vi "View Log Data.vi"() -> ()   [LabVIEW 2025]
uses:
  db86f9a9-b958-4c49-905b-a30c40e93e85.vi
  db86f9a9-b958-4c49-905b-a30c40e93e85.vi/4611cae3-c7be-41e2-9a5e-ea0ae78a7ced.vi
  db86f9a9-b958-4c49-905b-a30c40e93e85.vi/4611cae3-c7be-41e2-9a5e-ea0ae78a7ced.vi/19e2e4cb-e3bb-4239-bd5f-680916605f5d.vi
  db86f9a9-b958-4c49-905b-a30c40e93e85.vi/4611cae3-c7be-41e2-9a5e-ea0ae78a7ced.vi/f72612c1-738a-48a1-9fcf-3db66cb27fb3.vi
  db86f9a9-b958-4c49-905b-a30c40e93e85.vi/4611cae3-c7be-41e2-9a5e-ea0ae78a7ced.vi/45406051-8994-464b-8b47-ac12a8cbadfa.vi
  db86f9a9-b958-4c49-905b-a30c40e93e85.vi/4611cae3-c7be-41e2-9a5e-ea0ae78a7ced.vi/dd886480-778c-48b1-8e4a-d6890e1a60dd.vi
  db86f9a9-b958-4c49-905b-a30c40e93e85.vi/4611cae3-c7be-41e2-9a5e-ea0ae78a7ced.vi/2e6e140f-e361-4312-a09e-e37273ac7fd1.vi
  db86f9a9-b958-4c49-905b-a30c40e93e85.vi/4611cae3-c7be-41e2-9a5e-ea0ae78a7ced.vi/3589548e-4c68-4568-af05-72ab28470577.vi
  db86f9a9-b958-4c49-905b-a30c40e93e85.vi/4611cae3-c7be-41e2-9a5e-ea0ae78a7ced.vi/cf64d4f5-91bd-4749-9577-68c6ded0155b.vi
  db86f9a9-b958-4c49-905b-a30c40e93e85.vi/4611cae3-c7be-41e2-9a5e-ea0ae78a7ced.vi/6f6fefe9-f25b-4595-b26f-75715299a794.vi
  db86f9a9-b958-4c49-905b-a30c40e93e85.vi/4611cae3-c7be-41e2-9a5e-ea0ae78a7ced.vi/c74ffb76-1048-4639-9a95-b6de96ba7014.vi
panel:
  out "sorted array 3":T1(array[cluster])=[{"Particle Report"={"Area"=3719.0, "Number of Holes"=0.0, "Bounding Rect"={"Left"=1449.0, "Top"=174.0, "Right"=1530.0, "Bottom"=234.0}, "Center of Mass"={"X"=1488.0166711481581, "Y"=204.6493681097069}, "Orientation"=8.81828573662608, "Dimensions"={"Width"=81.0, "Height"=60.0}}, "angle"=-4.1875, "Distance"=2.981316858036219}]
  out "Image 2":T2(plugin-control)
  out "Image":T2(plugin-control)
  in  "index":i32
  out "Size":dbl=169.5
  in  "sorted array 2":T1(array[cluster])=[{"Particle Report"={"Area"=13014.0, "Number of Holes"=0.0, "Bounding Rect"={"Left"=1765.0, "Top"=174.0, "Right"=1928.0, "Bottom"=311.0}, "Center of Mass"={"X"=1850.7836944828646, "Y"=237.93722145381898}, "Orientation"=146.57468833541765, "Dimensions"={"Width"=163.0, "Height"=137.0}}, "angle"=40.4375, "Distance"=1.9142868762522598}]
  in  "Ring":u16(ring)=1 items=["2026-02-28 15:57:55", "2026-02-28 17:18:41"]
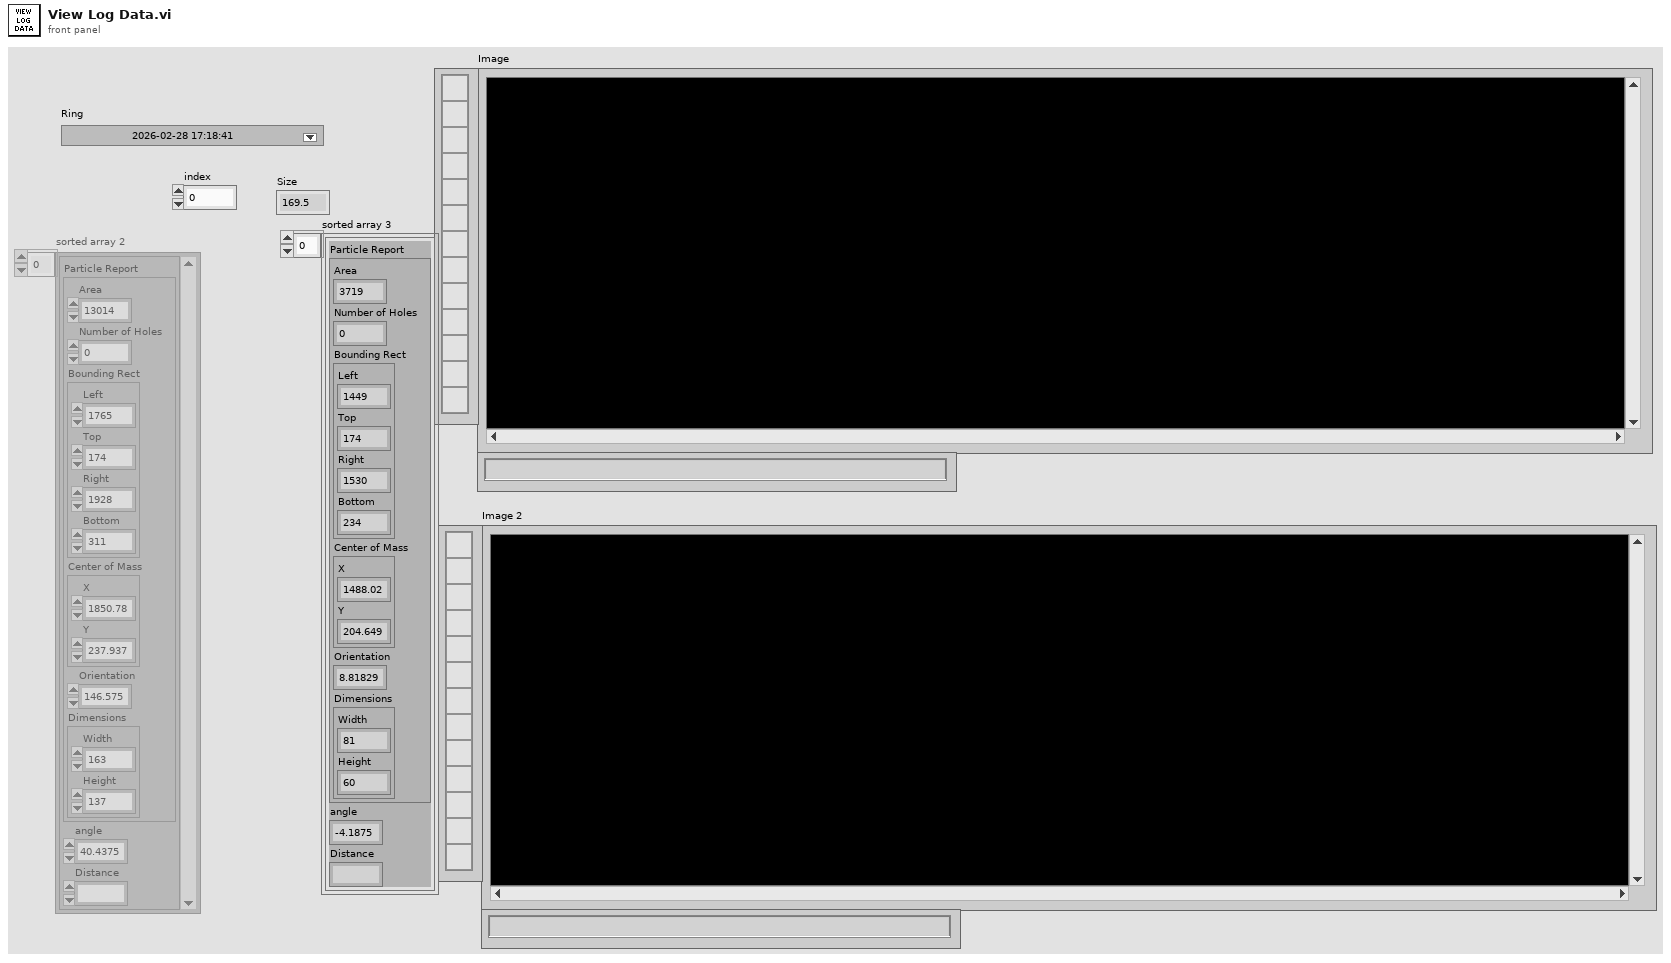
[diagram p1: front panel]
types:
  T1 = cluster{"Particle Report":cluster{"Area":dbl, "Number of Holes":dbl, "Bounding Rect":cluster{"Left":dbl, "Top":dbl, "Right":dbl, "Bottom":dbl}, "Center of Mass":cluster{"X":dbl, "Y":dbl}, "Orientation":dbl, "Dimensions":cluster{"Width":dbl, "Height":dbl}}, "angle":dbl, "Distance":ext}[]
  T2 = typedef "IMAQ Image.ctl" = refnum<image>
  T3 = typedef "Image Type" = u32
  T4 = cluster{"sorted array 2":cluster{"Particle Report":cluster{"Area":dbl, "Number of Holes":dbl, "Bounding Rect":cluster{"Left":dbl, "Top":dbl, "Right":dbl, "Bottom":dbl}, "Center of Mass":cluster{"X":dbl, "Y":dbl}, "Orientation":dbl, "Dimensions":cluster{"Width":dbl, "Height":dbl}}, "angle":dbl, "Distance":ext}[]}[]
  T5 = cluster{"sorted array 2":cluster{"Particle Report":cluster{"Area":dbl, "Number of Holes":dbl, "Bounding Rect":cluster{"Left":dbl, "Top":dbl, "Right":dbl, "Bottom":dbl}, "Center of Mass":cluster{"X":dbl, "Y":dbl}, "Orientation":dbl, "Dimensions":cluster{"Width":dbl, "Height":dbl}}, "angle":dbl, "Distance":ext}[]}
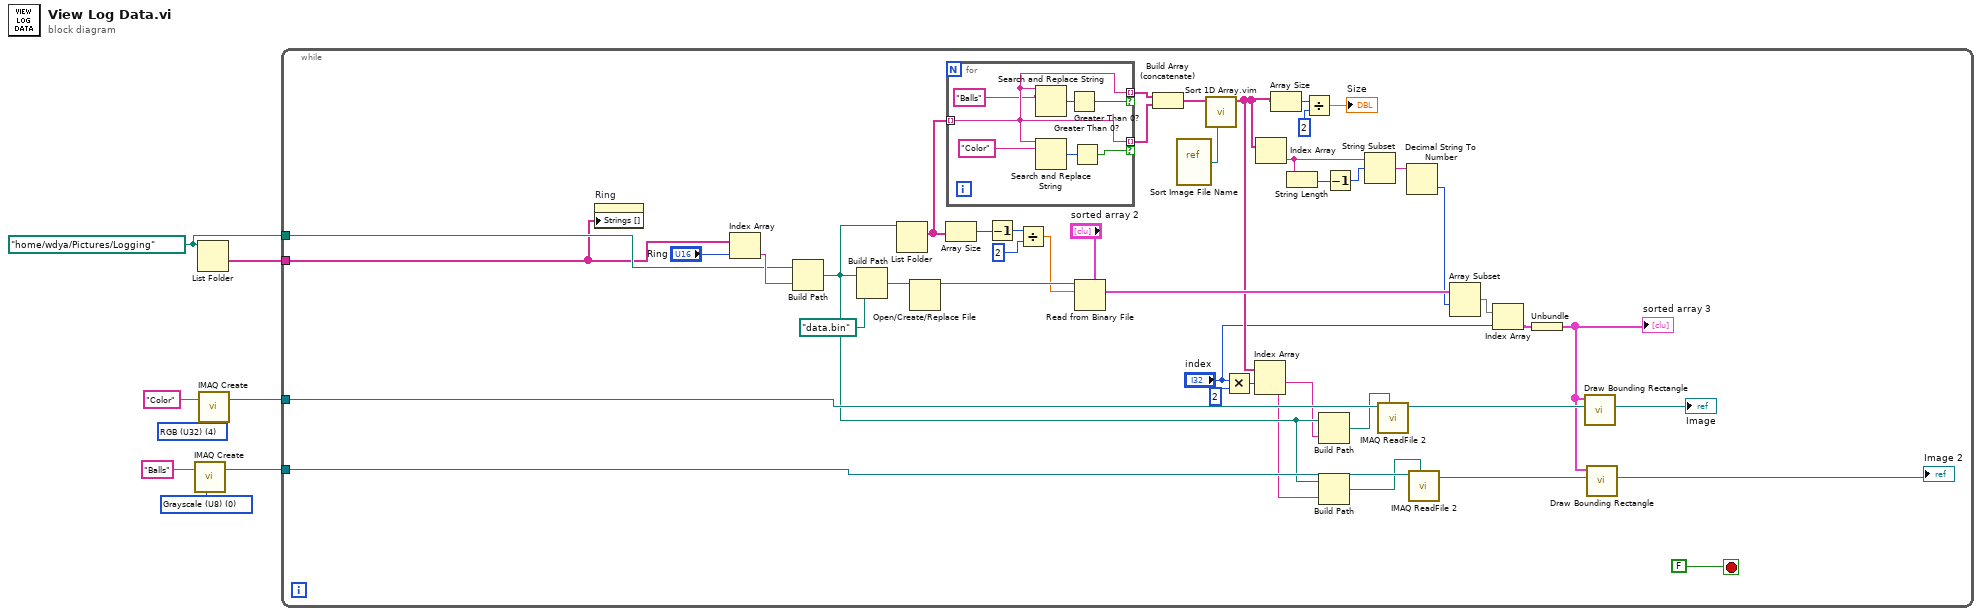
[diagram p0: block diagram]
diagram:
  w2 = path "/home/wdya/Pictures/Logging" ("path")
  w5 = T3 0 items=["Grayscale (U8)", "Grayscale (I16)", "Grayscale (SGL)", "Complex (CSG)", "RGB (U32)", "HSL (U32)", "RGB (U64)", "Grayscale (U16)"] ("Image Type")
  w7 = T3 4 items=["Grayscale (U8)", "Grayscale (I16)", "Grayscale (SGL)", "Complex (CSG)", "RGB (U32)", "HSL (U32)", "RGB (U64)", "Grayscale (U16)"] ("Image Type")
  n1 = call "IMAQ Create"("Image Name"="Balls", "Image Type"=w5) -> ("New Image"=w4:T2)  [unwired: 3 in, 1 out]
  n2 = List Folder(path=w2) -> (folder names=w1:string[])  [unwired: 3 in, 3 out]
  n3 = call "IMAQ Create"("Image Name"="Color", "Image Type"=w7) -> ("New Image"=w3:T2)  [unwired: 3 in, 1 out]
  n4 = while {
    tunnel: w4 -> [w29]
    tunnel: w3 -> [w28]
    tunnel: w2 -> [w13]
    tunnel: w1 -> [w12]
    stop <- FALSE stop-if-true
    n5 = property on="Ring" class="Ring (strict)"("Strings []"=w12) -> ()  [unwired: 2 in, 2 out]
    n6 = Index Array(array=w12, index="Ring") -> (element=w52:string)
    n7 = Build Path(base path=w13, name or relative path=w52) -> (appended path=w26:path)
    n8 = Build Path(base path=w26, name or relative path=path "data.bin" ("path")) -> (appended path=w48:path)
    n9 = List Folder(path=w26) -> (filenames=w43:string[])  [unwired: 3 in, 3 out]
    n10 = Open/Create/Replace File(file path (use dialog)=w48) -> (refnum out=w50:refnum<file>)  [unwired: 5 in, 2 out]
    n11 = Array Size(array=w43) -> (size(s)=w47:i32)
    n12 = for {
      tunnel: w43 -> [w60] mode=indexing
      tunnel: [w60] -> w41 mode=indexing if=w54
      tunnel: [w60] -> w42 mode=indexing if=w56
      n13 = Search and Replace String(input string=w60, search string="Balls") -> (number of replacements=w57:i32)  [unwired: 6 in, 3 out]
      n14 = Search and Replace String(input string=w60, search string="Color") -> (number of replacements=w55:i32)  [unwired: 6 in, 3 out]
      n15 = Greater Than 0?(x=w57) -> (x > 0?=w56:bool)
      n16 = Greater Than 0?(x=w55) -> (x > 0?=w54:bool)
    }
    n17 = Decrement(x=w47) -> (x-1=w46:i32)
    n18 = Divide(x=w46, y=2) -> (x/y=w44:dbl)
    n19 = Read from Binary File(5:"sorted array 2", 10:w44, 11:w50) -> (2:w36:T4)  [unwired: 3 in, 3 out]
    n20 = Build Array (concatenate)(w42, w41) -> (w39:string[])
    n21 = vi-ref "Sort Image File Name.vi"() -> (w40:refnum<vi>)
    n22 = call "Sort 1D Array.vim"("less function (built-in <)"=w40, "unsorted array"=w39) -> ("sorted array"=w27:string[])  [unwired: 9 in]
    n23 = Multiply(x="index", y=2) -> (x*y=w18:i32)
    n24 = Index Array(array=w27, index #1=w18) -> (element #1=w24:string, element #2=w25:string)  [unwired: 1 in]
    n25 = Index Array(array=w27) -> (element=w38:string)  [unwired: 1 in]
    n26 = Array Size(array=w27) -> (size(s)=w32:i32)
    n27 = String Length(string=w38) -> (length=w34:i32)
    n28 = Divide(x=w32, y=2) -> (x/y=→"Size":dbl)
    n29 = Build Path(base path=w26, name or relative path=w24) -> (appended path=w23:path)
    n30 = Build Path(base path=w26, name or relative path=w25) -> (appended path=w22:path)
    n31 = Decrement(x=w34) -> (x-1=w33:i32)
    n32 = String Subset(string=w38, offset (0)=w33) -> (substring=w37:string)  [unwired: 1 in]
    n33 = call "IMAQ ReadFile 2"("File Path"=w23, "Image"=w28) -> ("Image Out"=w15:T2)  [unwired: 5 in, 4 out]
    n34 = Decimal String To Number(string=w37) -> (number=w35:i32)  [unwired: 2 in, 1 out]
    n35 = call "IMAQ ReadFile 2"("File Path"=w22, "Image"=w29) -> ("Image Out"=w10:T2)  [unwired: 5 in, 4 out]
    n36 = Array Subset(array=w36, index=w35) -> (w21:T4)  [unwired: 1 in]
    n37 = Index Array(array=w21, index="index") -> (element=w16:T5)
    n38 = Unbundle(w16) -> ("sorted array 2"=w11:T1)
    "sorted array 3" <- w11
    n39 = call "Draw Bounding Rectangle.vi"("Image In"=w15, "sorted array"=w11) -> ("Image Out"=→"Image":T2)  [unwired: 8 in, 1 out]
    n40 = call "Draw Bounding Rectangle.vi"("Image In"=w10, "sorted array"=w11) -> ("Image Out"=→"Image 2":T2)  [unwired: 8 in, 1 out]
  }
